vi "Robot Turn (William + Michael S).vi"(7 "Reset":bool, 9 "X axis value":dbl, 10 "Desired Degree":dbl, 11 "Gyro Degrees":dbl) -> (3 "Stop":bool)   [LabVIEW 2014]
uses:
  Turn States.ctl
  <vilib>/Rock Robotics/WPI/RobotDrive/WPI_RobotDriveGetSetRefNum.vi
  <vilib>/Rock Robotics/WPI/RobotDrive/WPI_RobotDriveArcadeDrive_Standard(NoSaturation).vi
panel:
  out "Turn Right?":bool
  in  "Desired Time":dbl
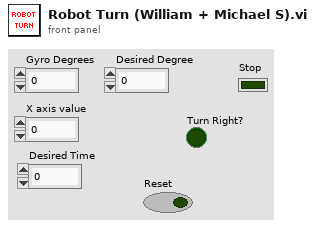
[diagram p1: front panel]
types:
  T1 = typedef "Turn States.ctl" = enum16{"Reset Encoder", "Determine Direction", "Turn Robot", "Stop"}
  T2 = typedef "WPI_GyroDevRef.ctl" = cluster{"DevStatus":errorcluster, "Analog Module":T3, "Analog Channel":T4, "Offset":dbl, "Gain (VoltsPerDegree/Second)":dbl}
  T3 = typedef "FPGA_TypedefAnalogModule.ctl" = enum16{"Controller 1"}
  T4 = typedef "FPGA_AIChannel.ctl" = enum8{"AI 0", "AI 1", "AI 2", "AI 3", "AI MXP 0", "AI MXP 1", "AI MXP 2", "AI MXP 3", "Invalid"}
  T5 = typedef "WPI_RobotDriveDevRef.ctl" = cluster{"DevStatus":errorcluster, "Motors[]":T6[], "Square Inputs":bool, "Max Output":dbl}
  T6 = typedef "WPI_MotorControlDeviceRef.ctl" = cluster{"DeviceStatus":errorcluster, "Type":T7, "PWM":cluster{"Controller":T8, "PWM Channel":T9, "DeadBand":T10}, "CAN":cluster{"Device Number":u8, "Control Mode":T11, "Semaphore":T12, "Max Vout":dbl, "TalonSRX Control Mode":T13}, "Invert":bool, "TransformRef":T14, "InvTransformRef":T14}
  T7 = typedef "WPI_MotorControlType.ctl" = enum16{"PWM", "CAN", "CANTalonSRX"}
  T8 = typedef "FPGA_TypedefDigitalModule.ctl" = enum16{"Controller 1"}
  T9 = typedef "FPGA_DIOPWMChannel.ctl" = enum8{"PWM 0", "PWM 1", "PWM 2", "PWM 3", "PWM 4", "PWM 5", "PWM 6", "PWM 7", "PWM 8", "PWM 9", "PWM MXP 0", "PWM MXP 1", "PWM MXP 2", "PWM MXP 3", "PWM MXP 4", "PWM MXP 5", "PWM MXP 6", "PWM MXP 7", "PWM MXP 8", "PWM MXP 9", "Invalid"}
  T10 = typedef "WPI_PWMDeadband.ctl" = cluster{"Name":string, "maxPositivePwm":i32, "minPositivePwm":i32, "centerPwm":i32, "maxNegativePwm":i32, "minNegativePwm":i32, "angularRange":u16}
  T11 = typedef "WPI_CANJaguar_ControlMode.ctl" = enum8{"Percent VBus", "Current", "Speed", "Position", "Voltage"}
  T12 = typedef "Semaphore RefNum" = refnum<k1>
  T13 = typedef "WPI_CANTalonSRX_APIControlMode.ctl" = enum8{"Percent VBus", "Speed", "Position", "Slave", "Unchanged / Invalid"}
  T14 = typedef "WPI_PWMTransform_ConPane.ctl" = refnum<vi>
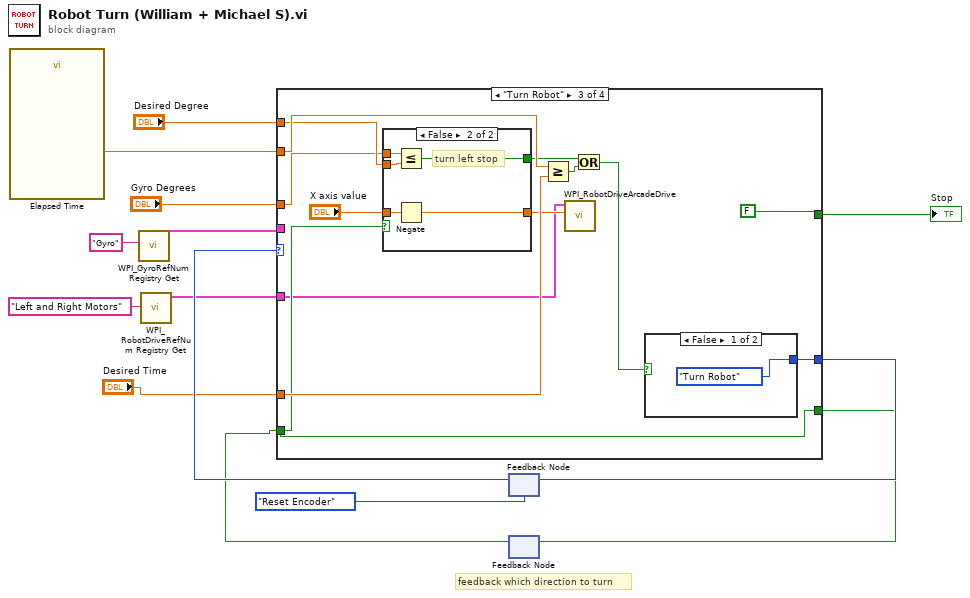
[diagram p0: block diagram]
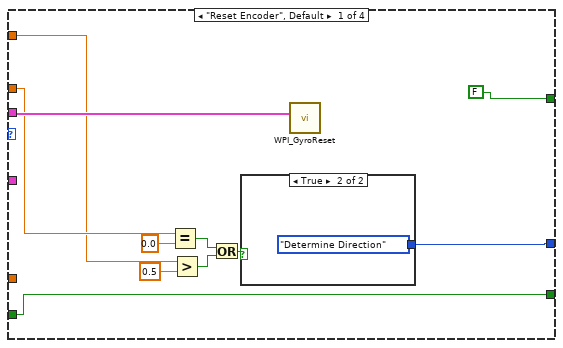
[diagram p2: hidden frame]
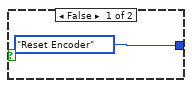
[diagram p3: hidden frame]
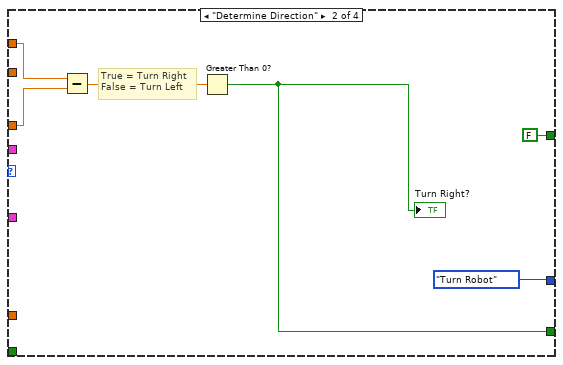
[diagram p4: hidden frame]
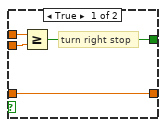
[diagram p5: hidden frame]
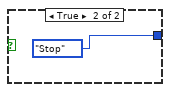
[diagram p6: hidden frame]
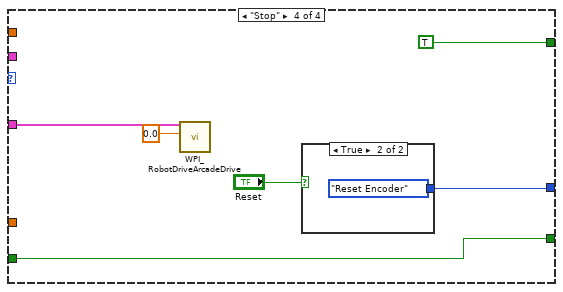
[diagram p7: hidden frame]
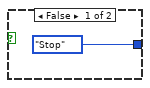
[diagram p8: hidden frame]
diagram:
  # "feedback which direction to turn"
  n1 = call "Elapsed Time"() -> ("Elapsed Time (s)"=w9:dbl)  [unwired: 12 in, 7 out]
  n2 = call <vilib>:"WPI_GyroRefNum Registry Get.vi"("refnum name"="Gyro") -> ("GyroDevRef"=w11:T2)  [unwired: 9 in, 1 out]
  n3 = call <vilib>:"WPI_RobotDriveRefNum Registry Get.vi"("refnum name"="Left and Right Motors") -> ("RobotDriveDevRef"=w6:T5)  [unwired: 9 in, 1 out]
  n4 = feedback #1(Turn_States."Reset Encoder") -> (w13:T1)
  n5 = feedback #2() -> (w1:bool)  [unwired: 1 in]
  n6 = case shown="\"Turn Robot\"" w13 {
    tunnel: w11 -> [w25 _ _ _]
    tunnel: "Gyro Degrees" -> [w24 w32 w39 _]
    tunnel: w9 -> [w22 _ w46 _]
    tunnel: [w18 Turn_States."Turn Robot" w43 w63] -> w8
    tunnel: w6 -> [_ _ w34 w58]
    tunnel: "Desired Degree" -> [_ w33 w40 _]
    tunnel: [FALSE FALSE FALSE TRUE] -> w4
    tunnel: "Desired Time" -> [_ _ w41 _]
    tunnel: [w15 w28 w35 w61] -> w2
    tunnel: w1 -> [w15 _ w35 w61]
    frame "Reset Encoder", Default {
      n7 = Equal?(x=w24, y=0.0) -> (x = y?=w20:bool)
      n8 = Greater?(x=w22, y=0.5) -> (0:w21:bool)
      n9 = Or(x=w20, y=w21) -> (x .or. y?=w19:bool)
      n10 = case shown="True" w19 {
        tunnel: [Turn_States."Reset Encoder" Turn_States."Determine Direction"] -> w18
        frame False {
        }
        frame True {
        }
      }
      n11 = call <vilib>:"WPI_GyroReset.vi"("GyroDevRef"=w25) -> ()  [unwired: 9 in, 2 out]
    }
    frame "Determine Direction" {
      # "True = Turn Right\nFalse = Turn Left"
      n12 = Subtract(x=w33, y=w32) -> (x-y=w31:dbl)
      n13 = Greater Than 0?(x=w31) -> (x > 0?=w28:bool)
      "Turn Right?" <- w28
    }
    frame "Turn Robot" {
      n14 = case shown="False" w35 {
        tunnel: w40 -> [w49 w54]
        tunnel: w39 -> [w50 w55]
        tunnel: [w48 w53] -> w38
        tunnel: "X axis value" -> [w47 w52]
        tunnel: [w47 w51] -> w36
        frame True {
          # "turn right stop"
          n15 = Greater Or Equal?(x=w50, y=w49) -> (x >= y?=w48:bool)
        }
        frame False {
          # "turn left stop"
          n16 = Less Or Equal?(x=w55, y=w54) -> (x <= y?=w53:bool)
          n17 = Negate(x=w52) -> (-x=w51:dbl)
        }
      }
      n18 = Greater Or Equal?(x=w46, y=w41) -> (x >= y?=w45:bool)
      n19 = call-poly <vilib>:"WPI_RobotDriveArcadeDrive.vi"("X axis value"=w36, "RobotDriveDevRef"=w34) -> ()  [unwired: 7 in, 3 out]
      n20 = Or(x=w38, y=w45) -> (x .or. y?=w44:bool)
      n21 = case shown="False" w44 {
        tunnel: [Turn_States."Turn Robot" Turn_States."Stop"] -> w43
        frame False {
        }
        frame True {
        }
      }
    }
    frame "Stop" {
      n22 = call-poly <vilib>:"WPI_RobotDriveArcadeDrive.vi"("X axis value"=0.0, "RobotDriveDevRef"=w58) -> ()  [unwired: 7 in, 3 out]
      n23 = case shown="True" "Reset" {
        tunnel: [Turn_States."Stop" Turn_States."Reset Encoder"] -> w63
        frame False {
        }
        frame True {
        }
      }
    }
  }
  "Stop" <- w4
  n24 = feedback-in #1(w8) -> ()
  n25 = feedback-in #2(w2) -> ()
